vi "ImageFilename.vi"(0 "Immediate":bool) -> (1 "Output Image Filename":string, 2 "TestImage":bool, 3 "Error":bool)   [LabVIEW 2014]
uses:
  globals/AzCamGlobals.vi
panel:
  in  "dir_remote":string caption="Directory"
  out "Remote image mode":bool
  in  "Image Format":T1(ring)
  in  "Rootname":string="itl."
  in  "Auto Name":bool
  out "Filename":string
  in  "dir_local":path=path "C:/data" caption="Directory"
  in  "Overwrite existing image":bool
  in  "Include sequence number":bool
  in  "Auto increment sequence":bool
  in  "Test Image":bool=TRUE
  in  "Close":bool
  in  "Sequence Number":i32=1 min=0 step=1
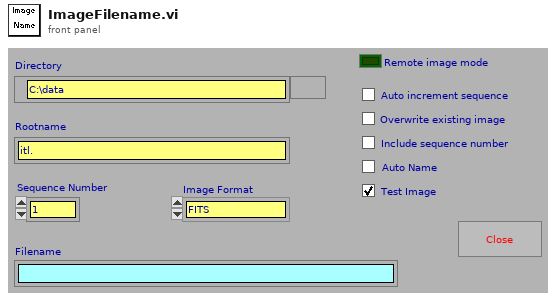
[diagram p1: front panel]
types:
  T1 = enum16{"FITS", "Extended FITS", "Binary", "TIFF", "JPEG", "GIF", "Thumbnail"}
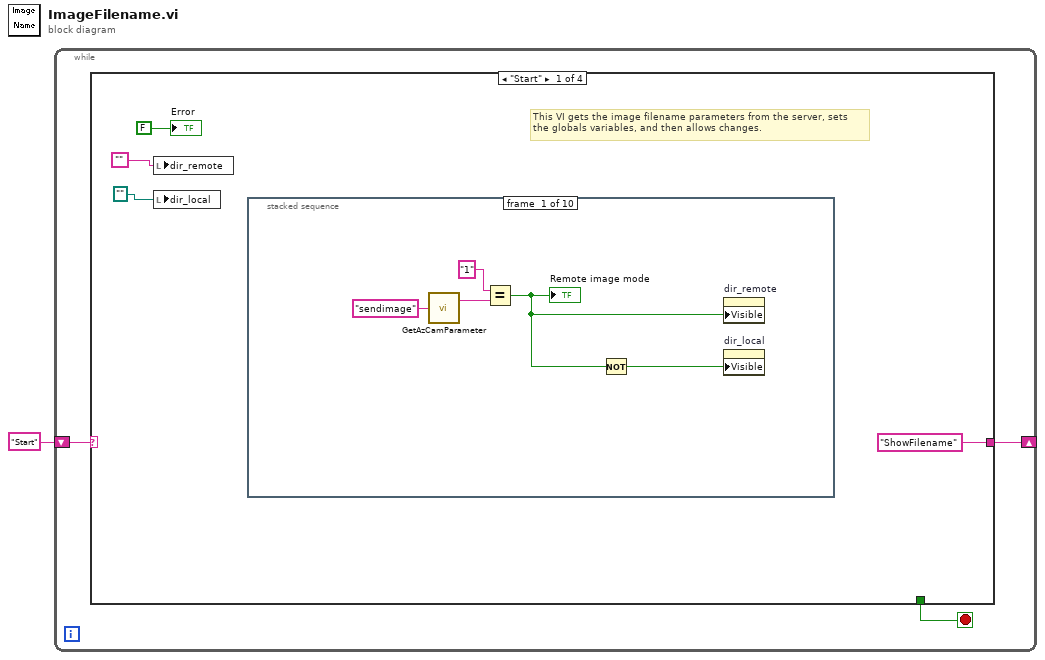
[diagram p0: block diagram]
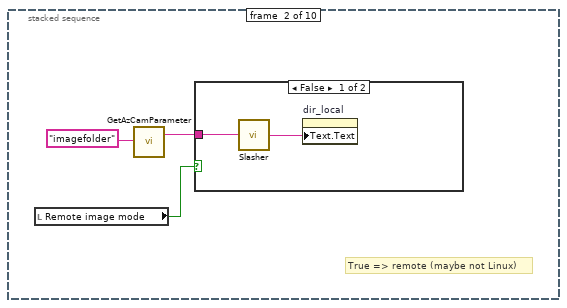
[diagram p2: hidden frame]
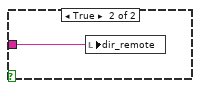
[diagram p3: hidden frame]
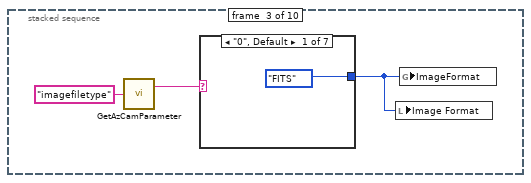
[diagram p4: hidden frame]
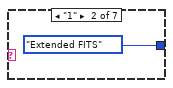
[diagram p5: hidden frame]
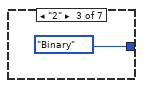
[diagram p6: hidden frame]
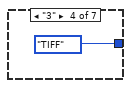
[diagram p7: hidden frame]
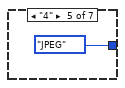
[diagram p8: hidden frame]
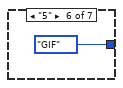
[diagram p9: hidden frame]
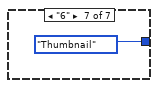
[diagram p10: hidden frame]
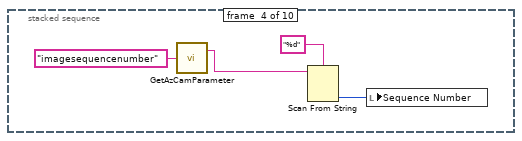
[diagram p11: hidden frame]
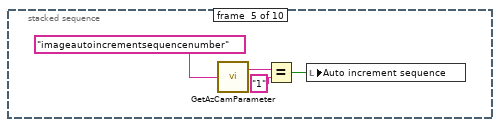
[diagram p12: hidden frame]
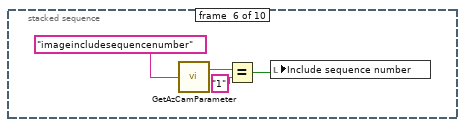
[diagram p13: hidden frame]
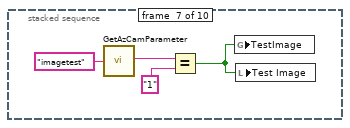
[diagram p14: hidden frame]
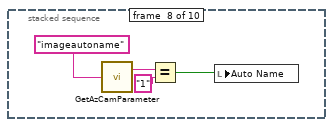
[diagram p15: hidden frame]
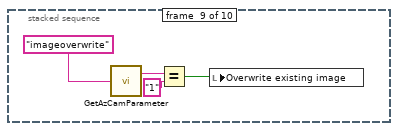
[diagram p16: hidden frame]
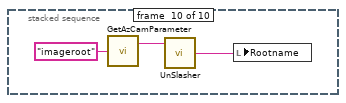
[diagram p17: hidden frame]
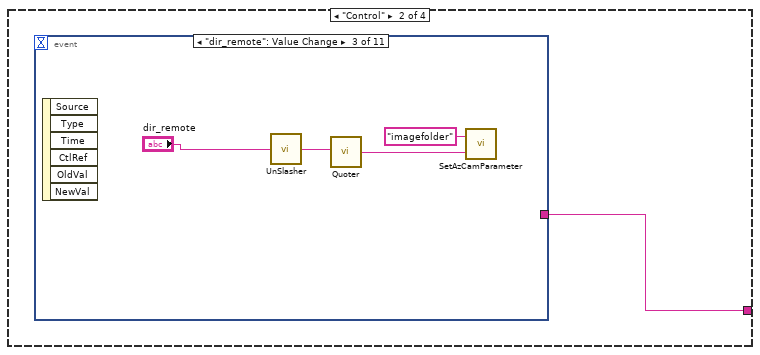
[diagram p18: hidden frame]
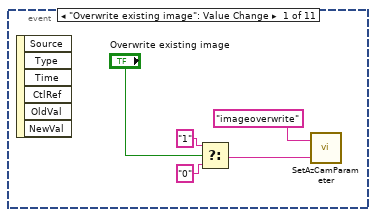
[diagram p19: hidden frame]
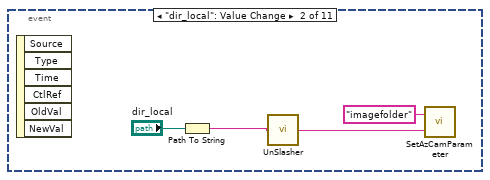
[diagram p20: hidden frame]
diagram:
  n1 = while {
    shift-right: [w2] -> _
    shift-left: "Start" -> [w3]
    stop <- w4 stop-if-true
    n2 = case shown="\"Start\"" w3 {
      tunnel: [_ _ _ TRUE] -> w4
      tunnel: ["ShowFilename" ("Rootname") w57 w117 _] -> w2
      frame "Start" {
        # "This VI gets the image filename parameters from the server, sets\nthe globals variables, and then allows changes."
        n3 = local write "dir_remote"("") -> ()
        n4 = local write "dir_local"(path "") -> ()
        n5 = stacked-sequence {
          frame #0 {
            n6 = call "GetAzCamParameter.vi"("Parameter"="sendimage") -> ("Value"=w12:string)  [unwired: 1 out]
            n7 = Equal?(x="1", y=w12) -> (x = y?=w9:bool)
            "Remote image mode" <- w9
            n8 = Not(x=w9) -> (.not. x?=w10:bool)
            n9 = property on="dir_remote" class="Str"("Visible"=w9) -> ()  [unwired: 2 in, 2 out]
            n10 = property on="dir_local" class="Path"("Visible"=w10) -> ()  [unwired: 2 in, 2 out]
          }
          frame #1 {
            # "True => remote (maybe not Linux)"
            n11 = local read "Remote image mode"() -> (w16:bool)
            n12 = call "GetAzCamParameter.vi"("Parameter"="imagefolder") -> ("Value"=w15:string)  [unwired: 1 out]
            n13 = case shown="False" w16 {
              tunnel: w15 -> [w18 w19]
              frame False {
                n14 = call "Slasher.vi"("String In"=w18) -> ("String Out"=w17:string)
                n15 = property on="dir_local" class="Path"("Text.Text"=w17) -> ()  [unwired: 2 in, 2 out]
              }
              frame True {
                n16 = local write "dir_remote"(w19) -> ()
              }
            }
          }
          frame #2 {
            n17 = call "GetAzCamParameter.vi"("Parameter"="imagefiletype") -> ("Value"=w20:string)  [unwired: 1 out]
            n18 = case shown="\"0\", Default" w20 {
              tunnel: [T1."FITS" ("ImageFormat") T1."Extended FITS" ("ImageFormat") T1."Binary" ("ImageFormat") T1."TIFF" ("ImageFormat") T1."JPEG" ("ImageFormat") T1."GIF" ("ImageFormat") T1."Thumbnail" ("ImageFormat")] -> w22
              frame "0", Default {
              }
              frame "1" {
              }
              frame "2" {
              }
              frame "3" {
              }
              frame "4" {
              }
              frame "5" {
              }
              frame "6" {
              }
            }
            n19 = local write "Image Format"(w22) -> ()
            n20 = global write "AzCamGlobals.vi" "ImageFormat"(w22) -> ()
          }
          frame #3 {
            n21 = call "GetAzCamParameter.vi"("Parameter"="imagesequencenumber") -> ("Value"=w30:string)  [unwired: 1 out]
            n22 = Scan From String(format string="%d", input string=w30) -> (output 1=w33:i32)  [unwired: 3 in, 3 out]
            n23 = local write "Sequence Number"(w33) -> ()
          }
          frame #4 {
            n24 = call "GetAzCamParameter.vi"("Parameter"="imageautoincrementsequencenumber") -> ("Value"=w36:string)  [unwired: 1 out]
            n25 = Equal?(x=w36, y="1") -> (x = y?=w34:bool)
            n26 = local write "Auto increment sequence"(w34) -> ()
          }
          frame #5 {
            n27 = call "GetAzCamParameter.vi"("Parameter"="imageincludesequencenumber") -> ("Value"=w40:string)  [unwired: 1 out]
            n28 = Equal?(x=w40, y="1") -> (x = y?=w38:bool)
            n29 = local write "Include sequence number"(w38) -> ()
          }
          frame #6 {
            n30 = call "GetAzCamParameter.vi"("Parameter"="imagetest") -> ("Value"=w42:string)  [unwired: 1 out]
            n31 = Equal?(x=w42, y="1") -> (x = y?=w44:bool)
            n32 = global write "AzCamGlobals.vi" "TestImage"(w44) -> ()
            n33 = local write "Test Image"(w44) -> ()
          }
          frame #7 {
            n34 = call "GetAzCamParameter.vi"("Parameter"="imageautoname") -> ("Value"=w48:string)  [unwired: 1 out]
            n35 = Equal?(x=w48, y="1") -> (x = y?=w46:bool)
            n36 = local write "Auto Name"(w46) -> ()
          }
          frame #8 {
            n37 = call "GetAzCamParameter.vi"("Parameter"="imageoverwrite") -> ("Value"=w53:string)  [unwired: 1 out]
            n38 = Equal?(x=w53, y="1") -> (x = y?=w51:bool)
            n39 = local write "Overwrite existing image"(w51) -> ()
          }
          frame #9 {
            n40 = call "GetAzCamParameter.vi"("Parameter"="imageroot") -> ("Value"=w55:string)  [unwired: 1 out]
            n41 = call "UnSlasher.vi"("String In"=w55) -> ("String Out"=w54:string)
            n42 = local write "Rootname"(w54) -> ()
          }
        }
        "Error" <- FALSE ("Error")
      }
      frame "Control" {
        n43 = event shown="[2] \"dir_remote\": Value Change" {
          selector: _ -> [_ _ _ _ _ _ _ _ _ _ _]
          dyn-events: _ -> [_ _ _ _ _ _ _ _ _ _ _]
          timeout: _ -> [_ _ _ _ _ _ _ _ _ _ _]
          tunnel: [_ _ _ _ _ _ "Control" _ _ _ "End"] -> w57
          event "Overwrite existing image": Value Change {
            n44 = event-data() -> ()  [unwired: 1 in, 6 out]
            n45 = Select(t="1", s="Overwrite existing image", f="0") -> (s? t:f=w58:string)
            n46 = call "SetAzCamParameter.vi"("Value"=w58, "Parameter"="imageoverwrite") -> ()  [unwired: 1 out]
          }
          event "dir_local": Value Change {
            n47 = event-data() -> ()  [unwired: 1 in, 6 out]
            n48 = Path To String(path="dir_local") -> (string=w64:string)
            n49 = call "UnSlasher.vi"("String In"=w64) -> ("String Out"=w63:string)
            n50 = call "SetAzCamParameter.vi"("Value"=w63, "Parameter"="imagefolder") -> ()  [unwired: 1 out]
          }
          event "dir_remote": Value Change {
            n51 = event-data() -> ()  [unwired: 1 in, 6 out]
            n52 = call "UnSlasher.vi"("String In"="dir_remote") -> ("String Out"=w67:string)
            n53 = call "Quoter.vi"("String In"=w67) -> ("String Out"=w69:string)
            n54 = call "SetAzCamParameter.vi"("Value"=w69, "Parameter"="imagefolder") -> ()  [unwired: 1 out]
          }
          event "Rootname": Value Change {
            n55 = event-data() -> ()  [unwired: 1 in, 6 out]
            n56 = call "Quoter.vi"("String In"="Rootname") -> ("String Out"=w71:string)
            n57 = call "SetAzCamParameter.vi"("Value"=w71, "Parameter"="imageroot") -> ()  [unwired: 1 out]
          }
          event "Sequence Number": Value Change {
            n58 = event-data() -> ()  [unwired: 1 in, 6 out]
            n59 = Format Into String(format string="%d", "Sequence Number") -> (resulting string=w74:string)  [unwired: 2 in, 1 out]
            n60 = call "SetAzCamParameter.vi"("Value"=w74, "Parameter"="imagesequencenumber") -> ()  [unwired: 1 out]
          }
          event "Image Format": Value Change {
            n61 = event-data() -> ()  [unwired: 1 in, 6 out]
            n62 = case shown="\"Extended FITS\"" "Image Format" {
              tunnel: ["0" ("Substring") "1" ("Substring") "2" ("Substring") "3" ("Substring") "4" ("Substring") "5" ("Substring") "6" ("Substring")] -> w78
              frame "FITS", Default {
              }
              frame "Extended FITS" {
              }
              frame "Binary" {
              }
              frame "TIFF" {
              }
              frame "JPEG" {
              }
              frame "GIF" {
              }
              frame "Thumbnail" {
              }
            }
            n63 = global write "AzCamGlobals.vi" "ImageFormat"("Image Format") -> ()
            n64 = call "SetAzCamParameter.vi"("Value"=w78, "Parameter"="imagefiletype") -> ()  [unwired: 1 out]
          }
          event "Auto increment sequence": Value Change {
            n65 = event-data() -> ()  [unwired: 1 in, 6 out]
            n66 = Select(t="1", s="Auto increment sequence", f="0") -> (s? t:f=w92:string)
            n67 = call "SetAzCamParameter.vi"("Value"=w92, "Parameter"="imageautoincrementsequencenumber") -> ()  [unwired: 1 out]
          }
          event "Include sequence number": Value Change {
            n68 = event-data() -> ()  [unwired: 1 in, 6 out]
            n69 = Select(t="1", s="Include sequence number", f="0") -> (s? t:f=w98:string)
            n70 = call "SetAzCamParameter.vi"("Value"=w98, "Parameter"="imageincludesequencenumber") -> ()  [unwired: 1 out]
          }
          event "Auto Name": Value Change {
            n71 = event-data() -> ()  [unwired: 1 in, 6 out]
            n72 = Select(t="1", s="Auto Name", f="0") -> (s? t:f=w103:string)
            n73 = call "SetAzCamParameter.vi"("Value"=w103, "Parameter"="imageautoname") -> ()  [unwired: 1 out]
          }
          event "Test Image": Value Change {
            n74 = event-data() -> ()  [unwired: 1 in, 6 out]
            n75 = global write "AzCamGlobals.vi" "TestImage"("Test Image") -> ()
            n76 = Select(t="1", s="Test Image", f="0") -> (s? t:f=w104:string)
            n77 = call "SetAzCamParameter.vi"("Value"=w104, "Parameter"="imagetest") -> ()  [unwired: 1 out]
          }
          event "Close": Value Change {
            n78 = event-data() -> ()  [unwired: 1 in, 6 out]
          }
        }
      }
      frame "ShowFilename", Default {
        n79 = call "GetAzCamParameter.vi"("Parameter"="imagefilename") -> ("Error"=w111:bool, "Value"=w110:string)
        "Filename" <- w110
        n80 = local write "Error"(w111) -> ()
        n81 = Search and Replace String(input string=w110, search string="\"") -> (result string=w113:string)  [unwired: 6 in, 3 out]
        "Output Image Filename" <- w113
        n82 = global write "AzCamGlobals.vi" "Filename"(w113) -> ()
        n83 = Select(t="End" ("Rootname"), s="Immediate", f="Control" ("Rootname")) -> (s? t:f=w117:string)
      }
      frame "End" {
        n84 = global read "AzCamGlobals.vi" "TestImage"() -> (→"TestImage":bool)
      }
    }
  }
